vi "Main.vi"() -> ()   [LabVIEW 2017, in "Bookmark Manager.lvlib"]
uses:
  Bookmark Manager.lvlib
  Private/Bookmarks Views.ctl
  Private/State.ctl
  Private/VI Bookmark.ctl
  Private/VI Information.ctl
  Private/Application Information.ctl
panel:
  in  "Bookmarks Filter":T1
  in  "Help":bool
  in  "Close":bool
  in  "Bookmarks":string(tree)
  in  "Scope":u16(ring) items=["Main Application Instance", "Eulogy.lvproj"]
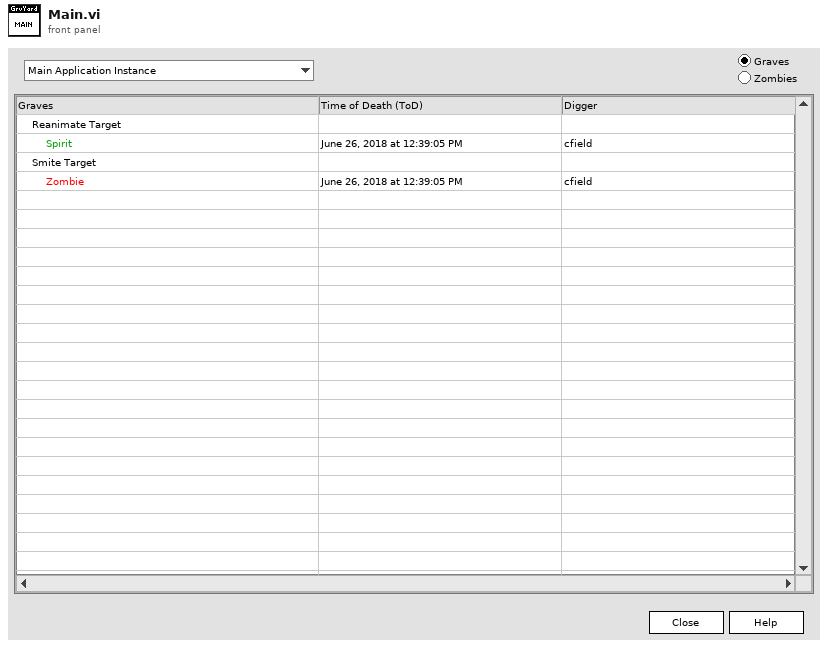
[diagram p1: front panel]
types:
  T1 = typedef "Bookmark Manager.lvlib/Bookmarks Views.ctl" = enum32{"Graves", "Zombies"}
  T2 = typedef "Bookmark Manager.lvlib/State.ctl" = cluster{"Bookmarks":T3[], "Bookmarks View":refnum<vi>, "Bookmarks Filter":T1, "Front Panel":refnum<vi>, "Scopes":refnum<vi>}
  T3 = typedef "Bookmark Manager.lvlib/VI Bookmark.ctl" = cluster{"Bookmark Info":cluster{"Bookmark ID":u32, "Bookmark Tag":string, "Label Text":string}, "VI Info":T4}
  T4 = typedef "Bookmark Manager.lvlib/VI Information.ctl" = cluster{"App Info":T5, "Name":string, "Path":path}
  T5 = typedef "Bookmark Manager.lvlib/Application Information.ctl" = cluster{"Project":string, "Target":string}
  T6 = enum32{"Invalid", "Standard", "Closed", "Hidden", "Minimized", "Maximized"}
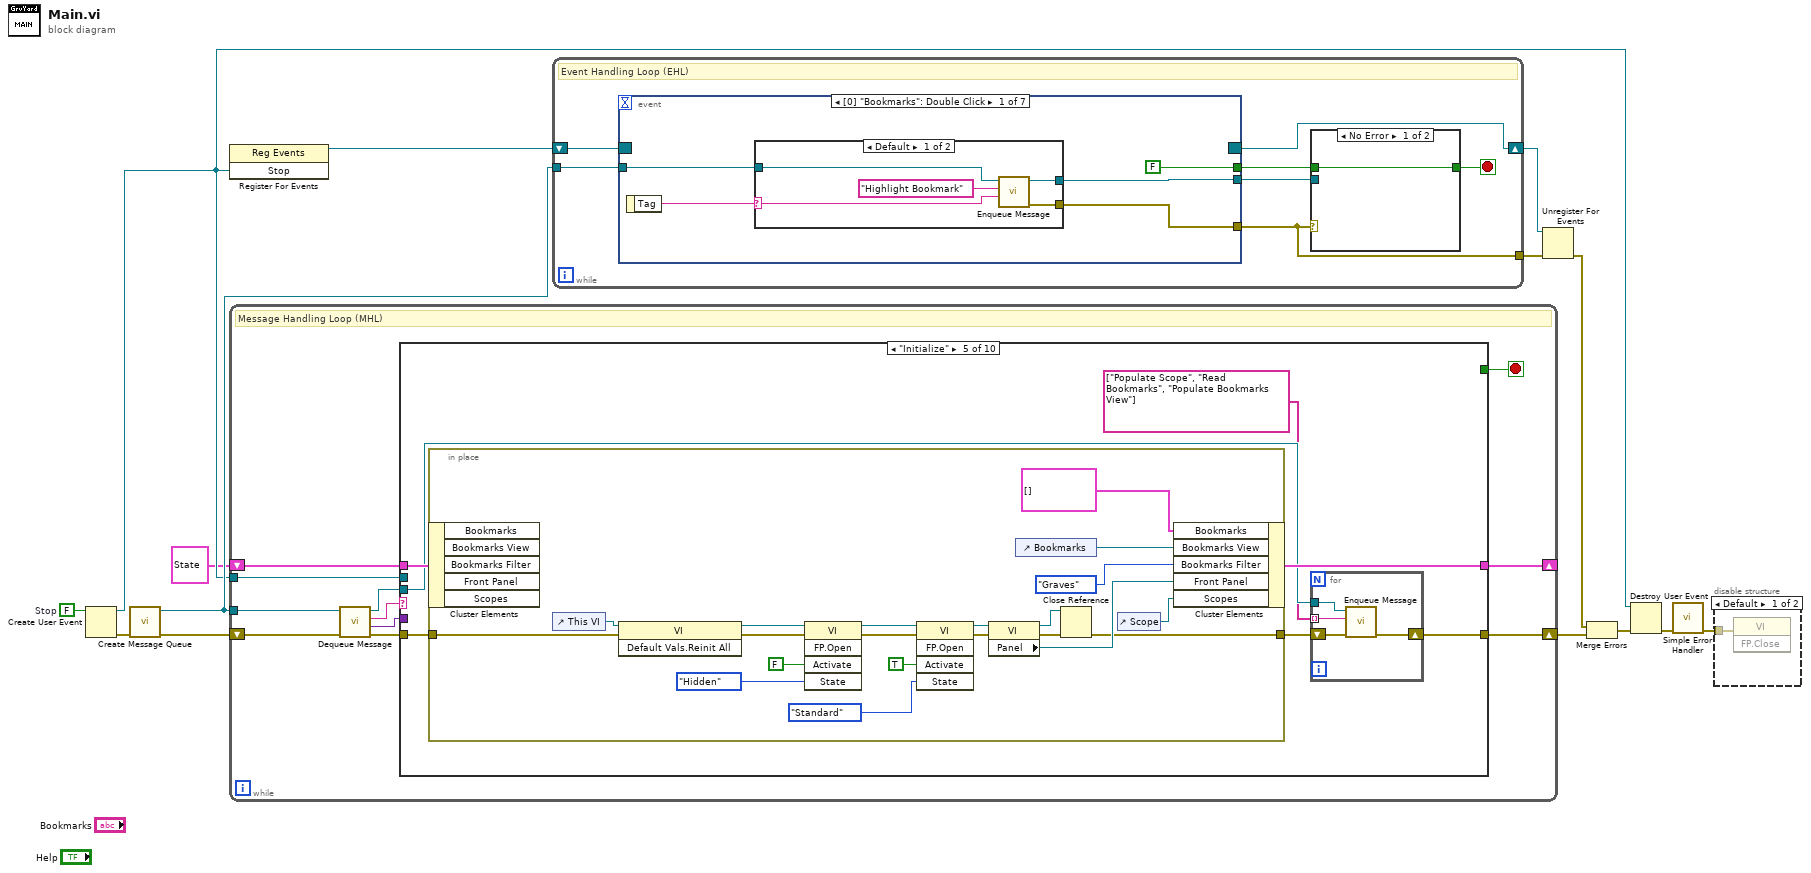
[diagram p0: block diagram]
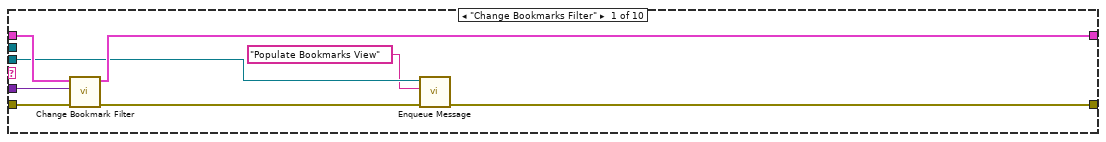
[diagram p3: hidden frame]
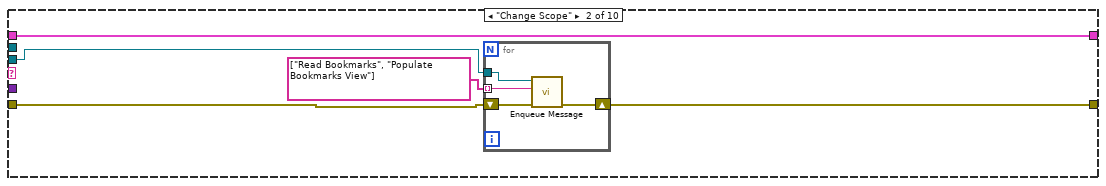
[diagram p4: hidden frame]
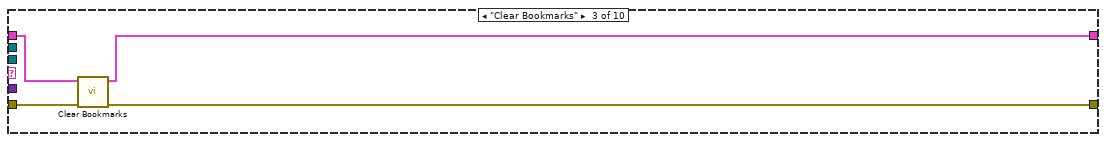
[diagram p5: hidden frame]
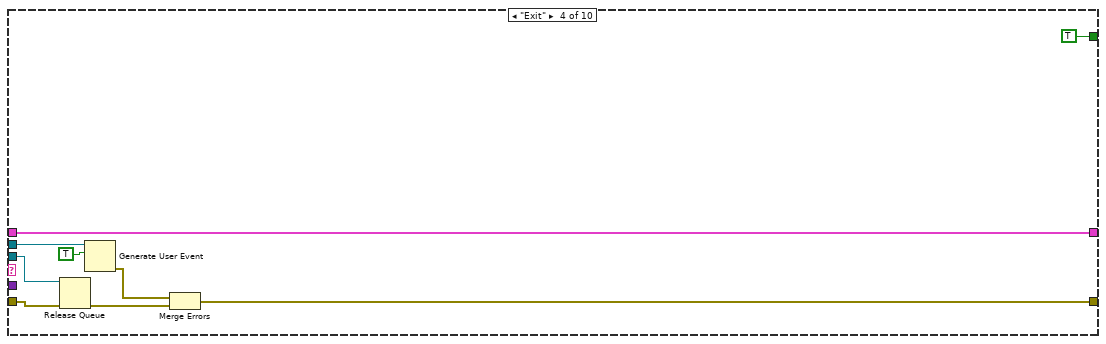
[diagram p6: hidden frame]
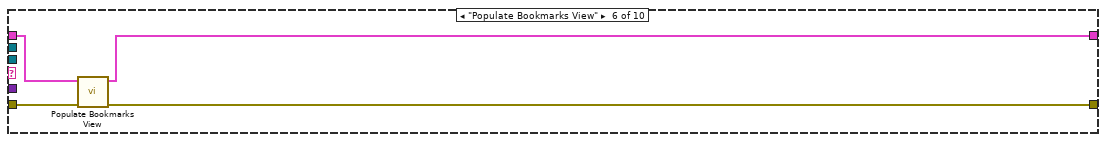
[diagram p7: hidden frame]
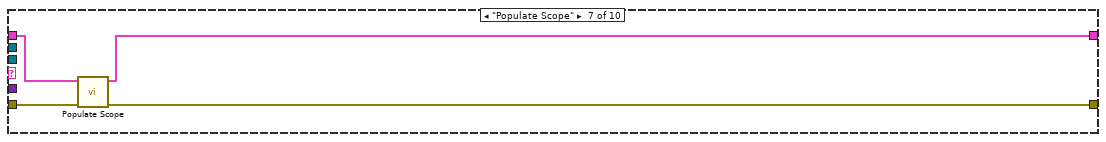
[diagram p8: hidden frame]
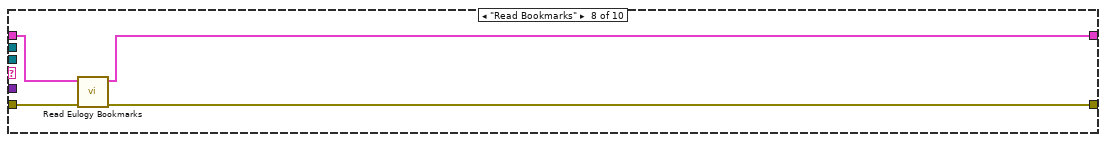
[diagram p9: hidden frame]
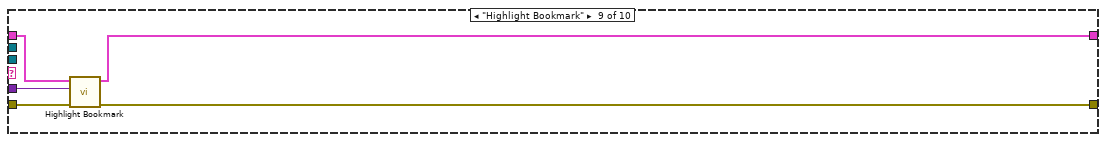
[diagram p10: hidden frame]
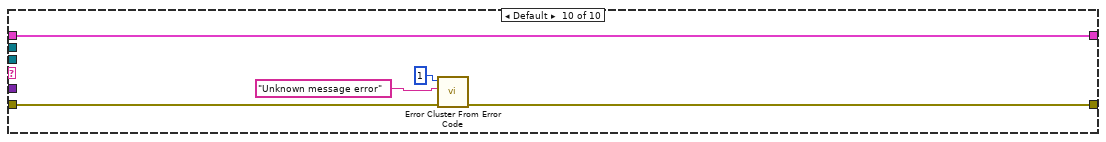
[diagram p11: hidden frame]
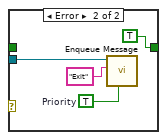
[diagram p12: hidden frame]
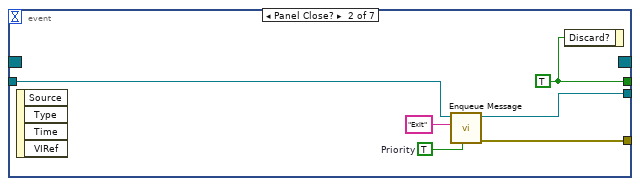
[diagram p14: hidden frame]
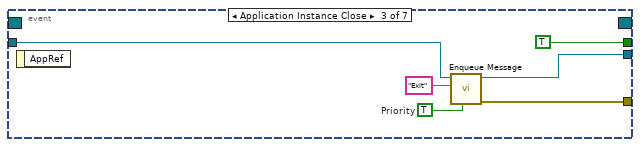
[diagram p15: hidden frame]
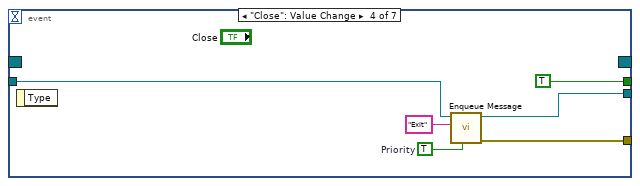
[diagram p16: hidden frame]
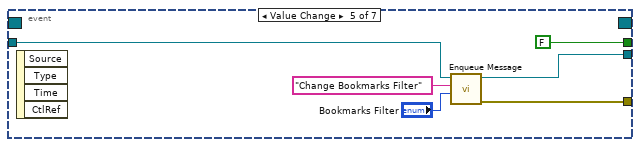
[diagram p17: hidden frame]
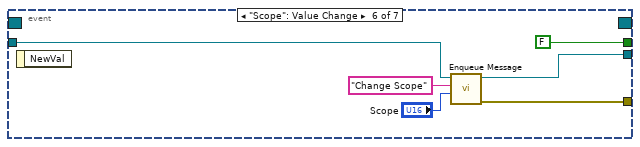
[diagram p18: hidden frame]
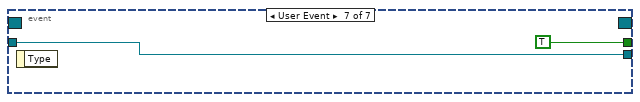
[diagram p19: hidden frame]
diagram:
  w11 = FALSE  # Stop
  n1 = Create User Event(user event datatype=w11) -> (user event=w4:refnum<user-event>, error out=w10:errorcluster)  [unwired: 1 in]
  n2 = call "Create Message Queue.vi"("Error In"=w10) -> ("Error Out"=w8:errorcluster, "Message Queue"=w9:refnum<queue>)  [unwired: 9 in]
  n3 = register-events(w4) -> (reference out=w14:refnum<event-registration>)  [unwired: 2 in, 1 out]
  n4 = while {
    tunnel: w9 -> [w25]
    shift-right: [w23] -> w6
    shift-left: w8 -> [w22]
    tunnel: w4 -> [w19]
    shift-right: [w16] -> _
    shift-left: T2 {"Bookmarks"=[], "Bookmarks View"=refnum, "Bookmarks Filter"=enum."Graves", "Front Panel"=refnum, "Scopes"=refnum} ("State") -> [w17]
    stop <- w20 stop-if-true
    # "Message Handling Loop (MHL)"
    n5 = call "Dequeue Message.vi"("Error In"=w22, "Message Queue In"=w25) -> ("Error Out"=w21:errorcluster, "Data"=w15:variant, "Command"=w24:string, "Message Queue Out"=w18:refnum<queue>)  [unwired: 6 in]
    n6 = case shown="\"Initialize\"" w24 {
      tunnel: [w28 w36 w43 w53 w57 w87 w91 w95 w100 w104] -> w23
      tunnel: w21 -> [w33 w38 w44 w55 w59 w88 w92 w96 w103 w106]
      tunnel: [_ _ _ TRUE _ _ _ _ _ _] -> w20
      tunnel: w19 -> [_ _ _ w52 _ _ _ _ _ _]
      tunnel: w18 -> [w27 w35 _ w48 w60 _ _ _ _ _]
      tunnel: w17 -> [w30 w37 w46 w47 w62 w90 w94 w98 w99 w105]
      tunnel: [w29 w37 w45 w47 w61 w89 w93 w97 w101 w105] -> w16
      tunnel: w15 -> [w31 _ _ _ _ _ _ _ w102 _]
      frame "Change Bookmarks Filter" {
        n7 = call "Change Bookmark Filter.vi"("Error In"=w33, "Data"=w31, "State In"=w30) -> ("Error Out"=w32:errorcluster, "State Out"=w29:T2)  [unwired: 7 in]
        n8 = call "Enqueue Message.vi"("Error In"=w32, "Command"="Populate Bookmarks View", "Message Queue In"=w27) -> ("Error Out"=w28:errorcluster)  [unwired: 7 in, 1 out]
      }
      frame "Change Scope" {
        n9 = for {
          tunnel: w35 -> [w40]
          tunnel: string[] ["Read Bookmarks", "Populate Bookmarks View"] -> [w39] mode=indexing
          shift-right: [w41] -> w36
          shift-left: w38 -> [w42]
          n10 = call "Enqueue Message.vi"("Error In"=w42, "Command"=w39, "Message Queue In"=w40) -> ("Error Out"=w41:errorcluster)  [unwired: 7 in, 1 out]
        }
      }
      frame "Clear Bookmarks" {
        n11 = call "Clear Bookmarks.vi"("Error In"=w44, "State In"=w46) -> ("Error Out"=w43:errorcluster, "State Out"=w45:T2)  [unwired: 8 in]
      }
      frame "Exit" {
        n12 = Release Queue(queue=w48, error in (no error)=w55) -> (error out=w49:errorcluster)  [unwired: 1 in, 2 out]
        n13 = Generate User Event(user event=w52, event data cluster=TRUE ("event data")) -> (error out=w50:errorcluster)  [unwired: 2 in, 1 out]
        n14 = Merge Errors(w50, w49) -> (w53:errorcluster)
      }
      frame "Initialize" {
        n15 = in-place {
          in-place-border: w59 -> [w82]
          in-place-border: [w78] -> w58
          n16 = in-place-cluster #1(w62) -> ()  [unwired: 5 out]
          n17 = control-ref of="This VI"() -> (w79:refnum<vi>)
          n18 = invoke class="VI" method="Default Vals.Reinit All"(reference=w79, error in=w82) -> (reference out=w81:refnum<vi>, error out=w70:errorcluster)  [unwired: 1 in, 1 out]
          n19 = invoke class="VI" method="FP.Open"(reference=w81, error in=w70, "Activate"=FALSE ("Activate?"), "State"=T6."Hidden") -> (reference out=w71:refnum<vi>, error out=w69:errorcluster)  [unwired: 1 in, 3 out]
          n20 = invoke class="VI" method="FP.Open"(reference=w71, error in=w69, "Activate"=TRUE ("Activate?"), "State"=T6."Standard") -> (reference out=w75:refnum<vi>, error out=w74:errorcluster)  [unwired: 1 in, 3 out]
          n21 = property class="VI"(reference=w75, error in=w74) -> (reference out=w77:refnum<vi>, error out=w80:errorcluster, "Panel"=w83:refnum<vi>)
          n22 = control-ref of="Bookmarks"() -> (w86:refnum<vi>)
          n23 = Close Reference(reference=w77, error in (no error)=w80) -> (error out=w78:errorcluster)
          n24 = control-ref of="Scope"() -> (w85:refnum<vi>)
          n25 = in-place-cluster #1("Bookmarks"=T3[] [], "Bookmarks View"=w86, "Bookmarks Filter"=Bookmarks_Views."Graves" ("Bookmarks Type"), "Front Panel"=w83, "Scopes"=w85) -> (w61:T2)
        }
        n26 = for {
          tunnel: w60 -> [w66]
          tunnel: string[] ["Populate Scope", "Read Bookmarks", "Populate Bookmarks View"] -> [w63] mode=indexing
          shift-right: [w64] -> w57
          shift-left: w58 -> [w65]
          n27 = call "Enqueue Message.vi"("Error In"=w65, "Command"=w63, "Message Queue In"=w66) -> ("Error Out"=w64:errorcluster)  [unwired: 7 in, 1 out]
        }
      }
      frame "Populate Bookmarks View" {
        n28 = call "Populate Bookmarks View.vi"("Error In"=w88, "State In"=w90) -> ("Error Out"=w87:errorcluster, "State Out"=w89:T2)  [unwired: 8 in]
      }
      frame "Populate Scope" {
        n29 = call "Populate Scope.vi"("Error In"=w92, "State In"=w94) -> ("Error Out"=w91:errorcluster, "State Out"=w93:T2)  [unwired: 8 in]
      }
      frame "Read Bookmarks" {
        n30 = call "Read Eulogy Bookmarks.vi"("Error In"=w96, "State In"=w98) -> ("Error Out"=w95:errorcluster, "State Out"=w97:T2)  [unwired: 8 in]
      }
      frame "Highlight Bookmark" {
        n31 = call "Highlight Bookmark.vi"("Error In"=w103, "Data"=w102, "State In"=w99) -> ("Error Out"=w100:errorcluster, "State Out"=w101:T2)  [unwired: 7 in]
      }
      frame Default {
        n32 = call <vilib>:"Error Cluster From Error Code.vi"("error in (no error)"=w106, "error message (\"\")"="Unknown message error" ("error message (\"\")"), "error code (0)"=1) -> ("error out"=w104:errorcluster)  [unwired: 6 in]
      }
    }
  }
  n33 = while {
    shift-right: [w114] -> w13
    shift-left: w14 -> [w115]
    tunnel: [w111] -> w12
    tunnel: w9 -> [w109]
    stop <- w112 stop-if-true
    # "Event Handling Loop (EHL)"
    n34 = event shown="[0] \"Bookmarks\": Double Click" {
      selector: w115 -> [_ _ _ _ _ _ _]
      dyn-events: [_ _ _ _ _ _ _] -> w114
      timeout: _ -> [_ _ _ _ _ _ _]
      tunnel: [w125 w135 w142 w148 w154 w160 _] -> w111
      tunnel: [FALSE w137 TRUE TRUE FALSE FALSE TRUE] -> w113
      tunnel: [w123 w136 w143 w149 w155 w161 w163] -> w110
      tunnel: w109 -> [w121 w132 w139 w145 w152 w159 w163]
      event "Bookmarks": Double Click {
        n35 = event-data() -> ("Tag"=w122:string)  [unwired: 1 in]
        n36 = case shown="Default" w122 {
          selector: w122 -> [w127 _]
          tunnel: [w129 _] -> w125
          tunnel: [w130 w131] -> w123
          tunnel: w121 -> [w126 w131]
          frame Default {
            n37 = call "Enqueue Message.vi"("Data"=w127, "Command"="Highlight Bookmark", "Message Queue In"=w126) -> ("Error Out"=w129:errorcluster, "Message Queue Out"=w130:refnum<queue>)  [unwired: 7 in]
          }
          frame "" {
          }
        }
      }
      event Panel Close? {
        w133 = TRUE  # Priority
        w137 = TRUE
        n38 = event-data() -> ()  [unwired: 1 in, 4 out]
        n39 = call "Enqueue Message.vi"("Priority"=w133, "Command"="Exit", "Message Queue In"=w132) -> ("Error Out"=w135:errorcluster, "Message Queue Out"=w136:refnum<queue>)  [unwired: 7 in]
        n40 = event-data("Discard?"=w137) -> ()  [unwired: 1 in, 1 out]
      }
      event Application Instance Close {
        w140 = TRUE  # Priority
        n41 = event-data() -> ()  [unwired: 1 in, 1 out]
        n42 = call "Enqueue Message.vi"("Priority"=w140, "Command"="Exit", "Message Queue In"=w139) -> ("Error Out"=w142:errorcluster, "Message Queue Out"=w143:refnum<queue>)  [unwired: 7 in]
      }
      event "Close": Value Change {
        w146 = TRUE  # Priority
        n43 = event-data() -> ()  [unwired: 1 in, 1 out]
        n44 = call "Enqueue Message.vi"("Priority"=w146, "Command"="Exit", "Message Queue In"=w145) -> ("Error Out"=w148:errorcluster, "Message Queue Out"=w149:refnum<queue>)  [unwired: 7 in]
      }
      event Value Change {
        n45 = event-data() -> ()  [unwired: 1 in, 4 out]
        n46 = call "Enqueue Message.vi"("Data"="Bookmarks Filter", "Command"="Change Bookmarks Filter", "Message Queue In"=w152) -> ("Error Out"=w154:errorcluster, "Message Queue Out"=w155:refnum<queue>)  [unwired: 7 in]
      }
      event "Scope": Value Change {
        n47 = event-data() -> ()  [unwired: 1 in, 1 out]
        n48 = call "Enqueue Message.vi"("Data"="Scope", "Command"="Change Scope", "Message Queue In"=w159) -> ("Error Out"=w160:errorcluster, "Message Queue Out"=w161:refnum<queue>)  [unwired: 7 in]
      }
      event User Event {
        n49 = event-data() -> ()  [unwired: 1 in, 1 out]
      }
    }
    n50 = case shown="No Error" w111 {
      tunnel: w113 -> [w116 _]
      tunnel: [w116 TRUE] -> w112
      tunnel: w110 -> [_ w119]
      frame No Error {
      }
      frame Error {
        w117 = TRUE  # Priority
        n51 = call "Enqueue Message.vi"("Priority"=w117, "Command"="Exit", "Message Queue In"=w119) -> ()  [unwired: 7 in, 2 out]
      }
    }
  }
  n52 = Unregister For Events(event registration refnum=w13, error in=w12) -> (error out=w7:errorcluster)
  n53 = Merge Errors(w7, w6) -> (w5:errorcluster)
  n54 = Destroy User Event(user event=w4, error in=w5) -> (error out=w3:errorcluster)
  n55 = call <vilib>:"Simple Error Handler.vi"("error in (no error)"=w3) -> ("error out"=w2:errorcluster)  [unwired: 4 in, 4 out]
  n56 = disable-structure shown="Default" {
    disable-tunnel: w2 -> [w164 _]
    frame condition #0 {
      n57 = invoke class="VI" method="FP.Close"(error in=w164) -> ()  [unwired: 2 in, 3 out]
    }
    frame condition #1 (active) {
    }
  }
